vi "Split Values into Channels.vi"(2 "values":u16[](array[numeric]), 3 "nOfChannels":u32) -> (1 "valuesPerChannel":u16[][](array[numeric]))   [LabVIEW 2016, in "pl1000.lvlib"]
doc: "Splits the a 1D array of values (output of GetValues) into a 2D array where each row represents a channel."
uses:
  pl1000.lvlib
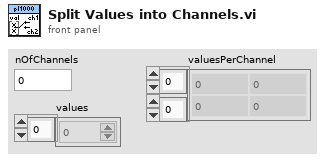
[diagram p1: front panel]
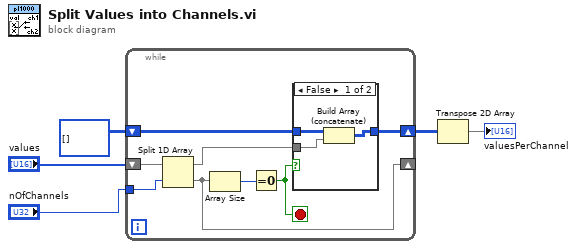
[diagram p0: block diagram]
diagram:
  n1 = while {
    tunnel: "nOfChannels" -> [w12]
    shift-right: [w10] -> _
    shift-left: "values" -> [w13]
    shift-right: [w7] -> w3
    shift-left: u16[][] [] -> [w9]
    stop <- w6 stop-if-true
    n2 = Split 1D Array(array=w13, index=w12) -> (first subarray=w8:u16[], second subarray=w10:u16[])
    n3 = Array Size(array=w10) -> (size(s)=w11:i32)
    n4 = Equal To 0?(x=w11) -> (x = 0?=w6:bool)
    n5 = case shown="False" w6 {
      tunnel: w9 -> [w16 w17]
      tunnel: w8 -> [w15 _]
      tunnel: [w14 w17] -> w7
      frame False {
        n6 = Build Array (concatenate)(w16, w15) -> (w14:u16[][])
      }
      frame True {
      }
    }
  }
  n7 = Transpose 2D Array(2D array=w3) -> (transposed array=→"valuesPerChannel":u16[][])
